vi "2L05-lambda_n0.vi"(5 "error in (no error)":errorcluster caption="err in", 6 "N(tfin)":u32, 7 "N(tdeb)":u32, 8 "tfin":dbl, 9 "tdeb":dbl) -> (3 "lambda":dbl, 4 "error out":errorcluster caption="err out")   [LabVIEW 2010, in "lv_02.lvlib"]
doc: "Calcul du taux de défaillance à partir d'une période de durée tdeb-tfin sur laquelle on dispose des effectifs en fonctionnement N(tdeb) et N(tfin) : Lambda = [N(tfin)-N(tdeb)] / [N(tdeb) * (tfin-tdeb) ]"
uses:
  lv_02.lvlib
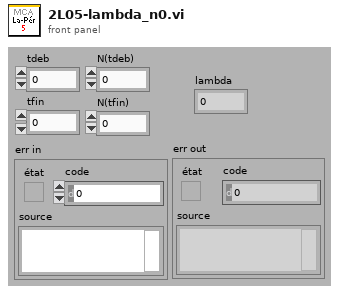
[diagram p1: front panel]
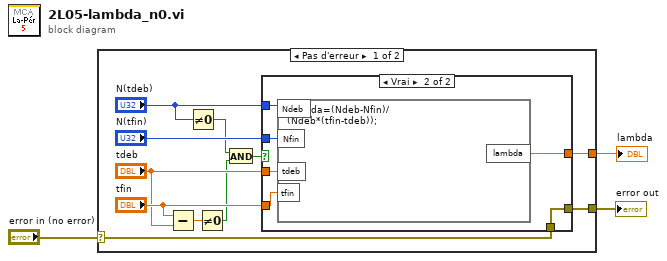
[diagram p0: block diagram]
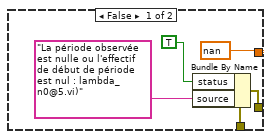
[diagram p2: hidden frame]
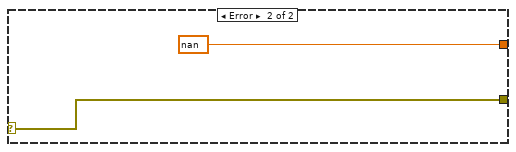
[diagram p3: hidden frame]
diagram:
  n1 = case shown="Pas d'erreur" "error in (no error)" {
    selector: "error in (no error)" -> [w6 w27]
    tunnel: [w5 w27] -> w2
    tunnel: [w4 nan ("lambda")] -> w1
    frame No Error {
      n2 = Subtract(x="tfin", y="tdeb") -> (x-y=w10:dbl)
      n3 = Not Equal To 0?(x="N(tdeb)") -> (x != 0?=w9:bool)
      n4 = Not Equal To 0?(x=w10) -> (x != 0?=w8:bool)
      n5 = And(x=w9, y=w8) -> (x .and. y?=w7:bool)
      n6 = case shown="Vrai" w7 {
        tunnel: "N(tfin)" -> [_ w25]
        tunnel: "N(tdeb)" -> [_ w24]
        tunnel: "tfin" -> [_ w20]
        tunnel: "tdeb" -> [_ w23]
        tunnel: [nan ("lambda") w22] -> w4
        tunnel: w6 -> [w18 w21]
        tunnel: [w15 w21] -> w5
        frame False {
          n7 = Bundle By Name(cluster=w18, "status"=TRUE, "source"="La période observée est nulle ou l'effectif de début de période est nul : lambda_n0@5.vi)") -> (w15:errorcluster)
        }
        frame True {
          n8 = formula code="lambda=(Ndeb-Nfin)/\n(Ndeb*(tfin-tdeb));"("tdeb"=w23, "Nfin"=w25, "Ndeb"=w24, "tfin"=w20) -> ("lambda"=w22:dbl)
        }
      }
    }
    frame Error {
    }
  }
  "error out" <- w2
  "lambda" <- w1
